vi "Gr to HR.vi"(1 "Grains [-]":dbl) -> (0 "Humidity Ratio [-]":dbl)   [LabVIEW 2020]
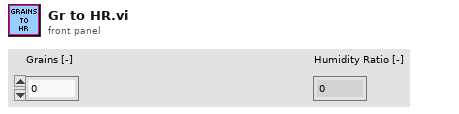
[diagram p1: front panel]
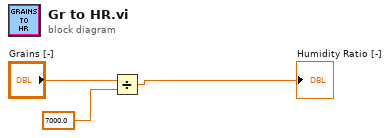
[diagram p0: block diagram]
diagram:
  n1 = Divide(x="Grains [-]", y=7000.0) -> (x/y=→"Humidity Ratio [-]":dbl)
